vi "Parameters3.vi"() -> ()   [LabVIEW 2018]
uses:
  Class 2.lvclass
panel:
  out "Udef 3":dbl
  out "Uinfl 3":dbl
  out "Ubender 3":dbl
  out "UIAT 3":dbl
  out "Uinj 3":dbl
  out "Im 3":dbl
  out "B0(T) 3":dbl
  out "B0(kGs) 3":dbl
  out "MeV/u 3":dbl
  out "F 3":dbl
  out "A/Z 3":dbl
  in  "Rm2":dbl
  out "Udef 2":dbl
  out "Uinfl 2":dbl
  out "Ubender 2":dbl
  out "UIAT 2":dbl
  out "Uinj 2":dbl
  out "Im 2":dbl
  out "B0(T) 2":dbl
  out "B0(kGs) 2":dbl
  out "MeV/u 2":dbl
  out "F 2":dbl
  out "A/Z 2":dbl
  in  "Rm":dbl
  out "Udef":dbl
  out "Uinfl":dbl
  out "Ubender":dbl
  out "UIAT":dbl
  out "Uinj":dbl
  out "Im":dbl
  out "B0(T)":dbl
  out "B0(kGs)":dbl
  out "MeV/u":dbl
  out "F":dbl
  in  "HARM":dbl=3.0
  out "A/Z":dbl
  in  "stop":bool
  in  "UECR":dbl
  in  "E (MeV)":dbl
  in  "Rextr":dbl=1.78
  in  "Z":dbl
  in  "A":dbl
  # "Инфлектор типа A"
  # "14N3+"
  # "Инфлектор типа B"
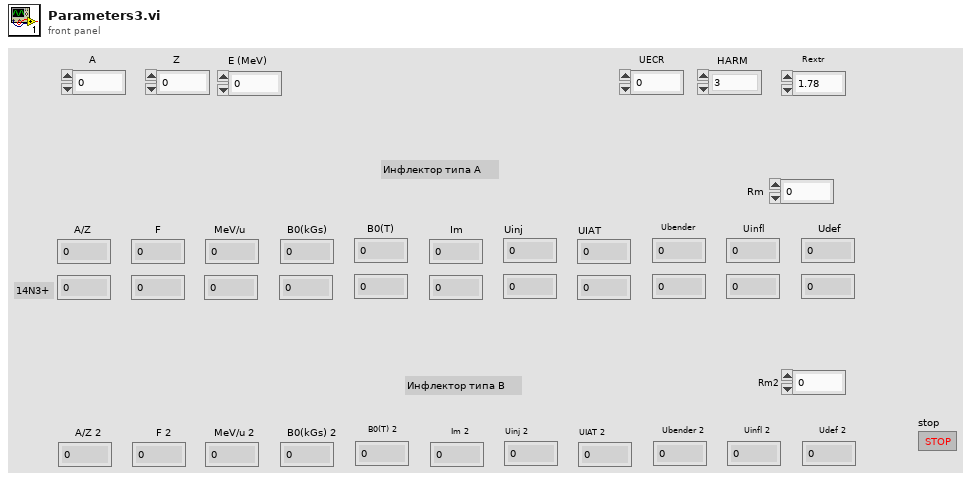
[diagram p1: front panel]
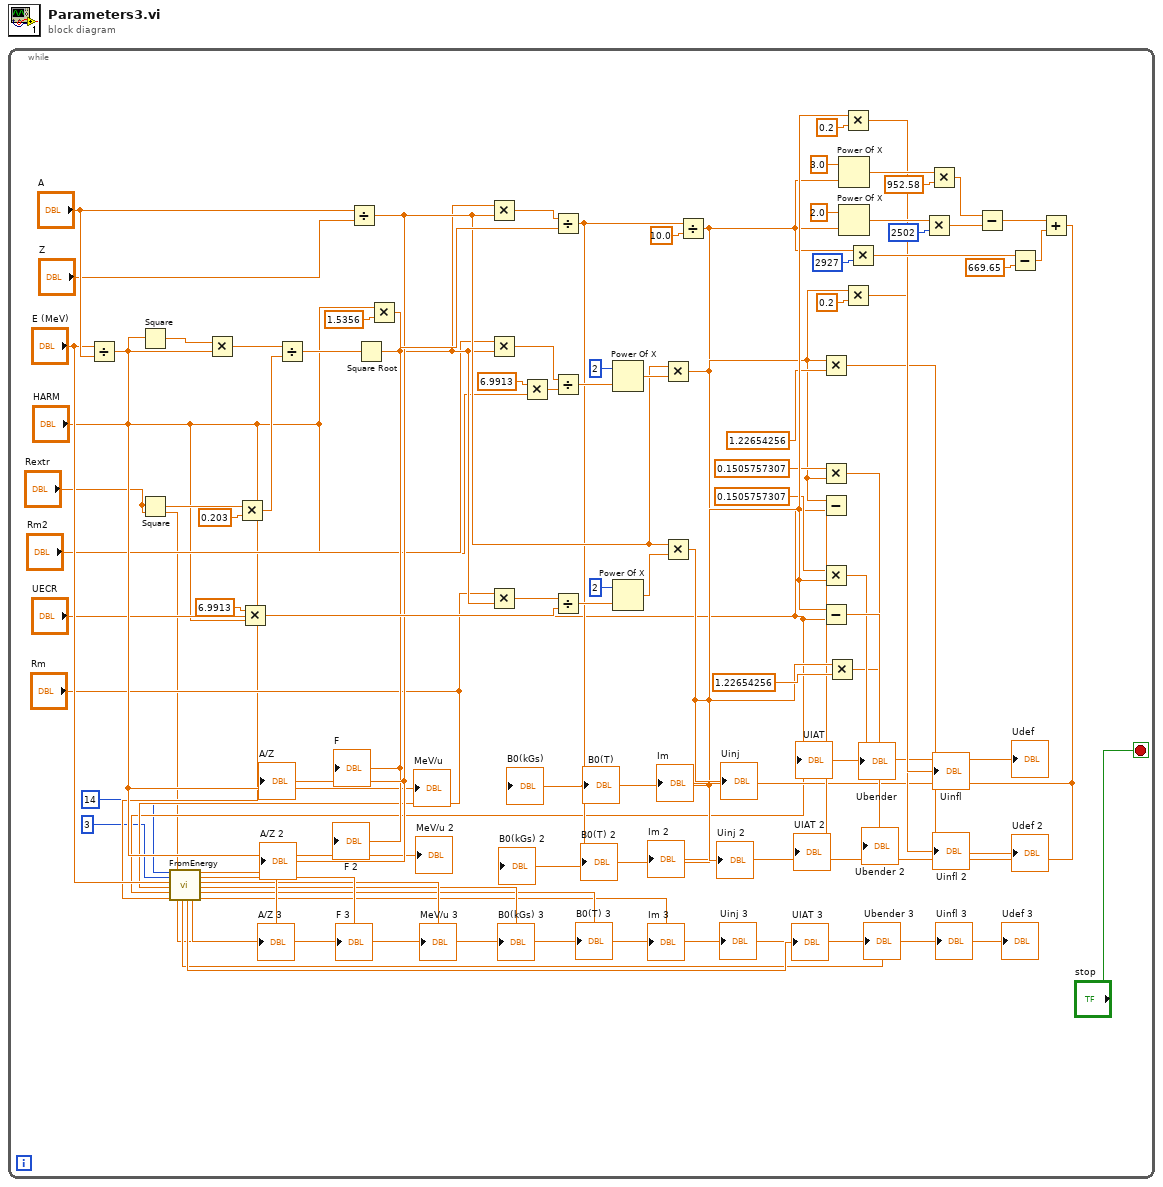
[diagram p0: block diagram]
diagram:
  n1 = while {
    stop <- "stop" stop-if-true
    n2 = Divide(x="E (MeV)", y="A") -> (x/y=w23:dbl)
    "MeV/u" <- w23
    "MeV/u 2" <- w23
    n3 = Square(x="HARM") -> (x^2=w78:dbl)
    n4 = Square(x="Rextr") -> (x^2=w77:dbl)
    n5 = call "FromEnergy.vi"("A"=14, "Z"=3, "E (MeV)"="E (MeV)", "Rm"="Rm", "UECR"="UECR", "HARM"="HARM", "Rextr"="Rextr") -> ("Uinfl"=→"Uinfl 3":dbl, "Ubender"=→"Ubender 3":dbl, "UIAT"=→"UIAT 3":dbl, "Udef"=→"Udef 3":dbl, "Uinj"=→"Uinj 3":dbl, "A/Z"=→"A/Z 3":dbl, "F"=→"F 3":dbl, "MeV/u"=→"MeV/u 3":dbl, "B0(kGs)"=→"B0(kGs) 3":dbl, "B0(T)"=→"B0(T) 3":dbl, "Im"=→"Im 3":dbl)  [unwired: 2 in]
    n6 = Multiply(x=w78, y=w23) -> (x*y=w75:dbl)
    n7 = Multiply(x=w77, y=0.203) -> (x*y=w74:dbl)
    n8 = Multiply(x=6.9913, y="HARM") -> (x*y=w53:dbl)
    n9 = Divide(x=w75, y=w74) -> (x/y=w73:dbl)
    n10 = Divide(x="A", y="Z") -> (x/y=w27:dbl)
    "A/Z" <- w27
    "A/Z 2" <- w27
    n11 = Square Root(x=w73) -> (sqrt(x)=w26:dbl)
    "F" <- w26
    "F 2" <- w26
    n12 = Multiply(x="HARM", y=1.5356) -> (x*y=w70:dbl)
    n13 = Multiply(x=w26, y=w27) -> (x*y=w71:dbl)
    n14 = Multiply(x="Rm2", y=w26) -> (x*y=w41:dbl)
    n15 = Multiply(x="Rm", y=w26) -> (x*y=w54:dbl)
    n16 = Multiply(x=6.9913, y="HARM") -> (x*y=w40:dbl)
    n17 = Divide(x=w71, y=w70) -> (x/y=w24:dbl)
    "B0(kGs)" <- w24
    "B0(kGs) 2" <- w24
    n18 = Divide(x=w41, y=w40) -> (x/y=w39:dbl)
    n19 = Divide(x=w54, y=w53) -> (x/y=w52:dbl)
    n20 = Power Of X(1:w39, 2:2) -> (0:w37:dbl)
    n21 = Power Of X(1:w52, 2:2) -> (0:w50:dbl)
    n22 = Multiply(x=w27, y=w37) -> (x*y=w32:dbl)
    "Uinj 2" <- w32
    n23 = Multiply(x=w27, y=w50) -> (x*y=w43:dbl)
    "Uinj" <- w43
    n24 = Divide(x=w24, y=10.0) -> (x/y=w25:dbl)
    "B0(T)" <- w25
    "B0(T) 2" <- w25
    n25 = Multiply(x=w32, y=1.22654256) -> (x*y=→"Udef 2":dbl)
    n26 = Multiply(x=0.1505757307, y=w32) -> (x*y=→"Ubender 2":dbl)
    n27 = Subtract(x=w32, y="UECR") -> (x-y=→"UIAT 2":dbl)
    n28 = Multiply(x=0.1505757307, y=w43) -> (x*y=→"Ubender":dbl)
    n29 = Subtract(x=w43, y="UECR") -> (x-y=→"UIAT":dbl)
    n30 = Multiply(x=w43, y=1.22654256) -> (x*y=→"Udef":dbl)
    n31 = Power Of X(1:w25, 2:3.0 ("y")) -> (0:w67:dbl)
    n32 = Power Of X(1:w25, 2:2.0 ("y")) -> (0:w65:dbl)
    n33 = Multiply(x=w43, y=0.2) -> (x*y=→"Uinfl":dbl)
    n34 = Multiply(x=w32, y=0.2) -> (x*y=→"Uinfl 2":dbl)
    n35 = Multiply(x=w25, y=2927) -> (x*y=w59:dbl)
    n36 = Multiply(x=w65, y=2502) -> (x*y=w60:dbl)
    n37 = Multiply(x=w67, y=952.58) -> (x*y=w61:dbl)
    n38 = Subtract(x=w61, y=w60) -> (x-y=w57:dbl)
    n39 = Subtract(x=w59, y=669.65) -> (x-y=w56:dbl)
    n40 = Add(x=w57, y=w56) -> (x+y=→"Im" →"Im 2":dbl)
  }
